vi "Get Mutation History - NONUI.vi"(6 "error in":errorcluster, 9 "Input object":refnum<class>) -> (0 "error out":errorcluster, 1 "Mutation History":T1 {"LabVIEW Version" format="%.0x"})   [LabVIEW 2019, in "IncrementMutationHistory.lvlib" / "VILIB_NONUI.lvlib"]
doc: "A mutation history is a record of all the version changes that a class has undergone and a recipie for converting flattened data of the old versions into the new version of the class. Each LabVIEW class stores its own mutation history and the mutation history for all of its ancestors. All of the mutation histories that a class records are collectively called its geneology. \n\nThis VI allows you to get a copy of the mutation history for the class or any of its ancestors. The input object is the class whose geneology you wish to search. The class name input is the mutation history that you want to find."
uses:
  <vilib>/Utility/EditLVLibs/LVClass/Mutation History.ctl
  <vilib>/Utility/EditLVLibs/LVClass/Mutation Record.ctl
  <vilib>/Utility/EditLVLibs/LibVersion.ctl
  VILIB_NONUI.lvlib
  <vilib>/Utility/EditLVLibs/Edit LVLibs.lvlib
panel:
  in  "error message 2":string="LabVIEW Object does not have mutation history for any class."
  in  "error message 1":string="The class library of the input object does not have any mutation history."
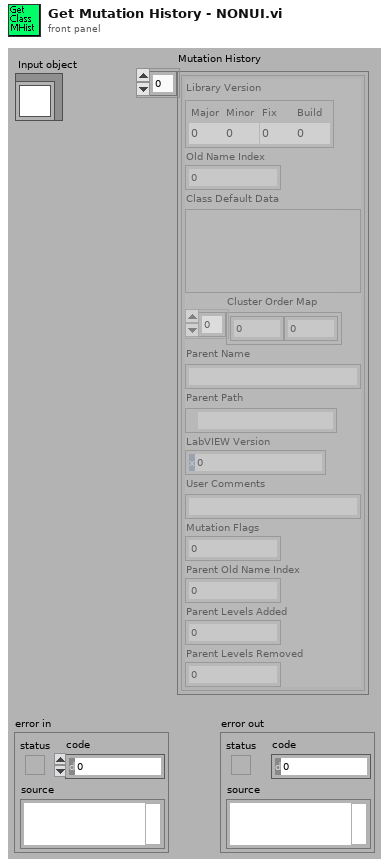
[diagram p1: front panel]
types:
  T1 = typedef "Edit LVLibs.lvlib/Mutation History.ctl" = T2[]
  T2 = typedef "Edit LVLibs.lvlib/Mutation Record.ctl" = cluster{"Library Version":T3, "Old Name Index":u8, "Class Default Data":variant, "Cluster Order Map":u32[], "Parent Name":string, "Parent Path":path, "LabVIEW Version":u32, "User Comments":string, "Mutation Flags":u8, "Parent Old Name Index":u8, "Parent Levels Added":u16, "Parent Levels Removed":u16}
  T3 = typedef "Edit LVLibs.lvlib/LibVersion.ctl" = cluster{"Major":u16, "Minor":u16, "Fix":u16, "Build":u16}
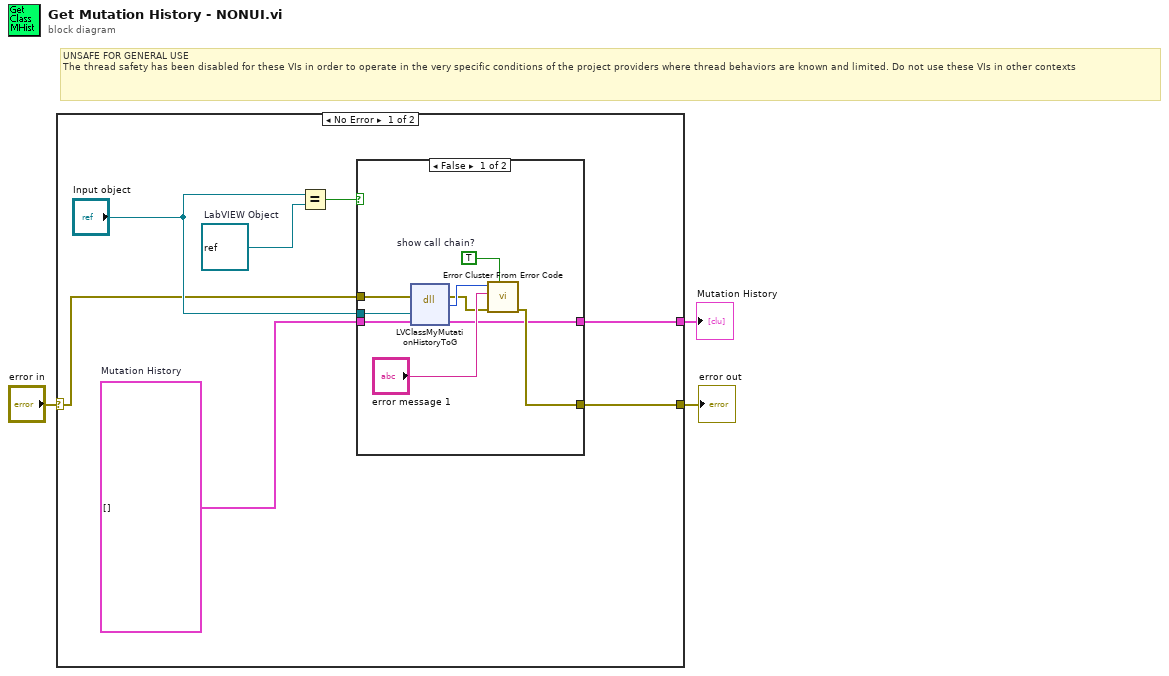
[diagram p0: block diagram]
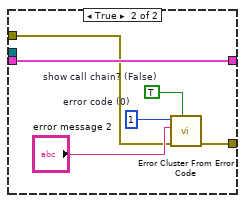
[diagram p2: hidden frame]
diagram:
  # "UNSAFE FOR GENERAL USE\nThe thread safety has been disabled for these VIs in order to operate in the very specific conditions of the project providers where thread behaviors are known and limited. Do not use these VIs in other contexts"
  n1 = case shown="No Error" "error in" {
    selector: "error in" -> [w4 w26]
    tunnel: [w7 w26] -> w3
    tunnel: [w6 _] -> w1
    frame No Error {
      w5 = refnum<class> refnum  # LabVIEW Object
      w10 = T1 []  # Mutation History
      n2 = Equal?(x="Input object", y=w5) -> (x = y?=w8:bool)
      n3 = case shown="False" w8 {
        tunnel: w10 -> [w15 w25]
        tunnel: [w14 w25] -> w6
        tunnel: "Input object" -> [w16 _]
        tunnel: [w17 w21] -> w7
        tunnel: w4 -> [w11 w20]
        frame False {
          w19 = TRUE  # show call chain?
          n4 = dll-call lib="LabVIEW" fn="LVClassMyMutationHistoryToG"(error in=w11, "object"=w16, "mutation records"=w15) -> (error out=w12:errorcluster, "return type"=w13:i32, "mutation records"=w14:T1)  [unwired: 3 in, 1 out]
          n5 = call <vilib>:"Error Cluster From Error Code.vi"("show call chain? (False)"=w19, "error in (no error)"=w12, "error message (\"\")"="error message 1", "error code (0)"=w13) -> ("error out"=w17:errorcluster)  [unwired: 5 in]
        }
        frame True {
          w23 = 1  # error code (0)
          w24 = TRUE  # show call chain? (False)
          n6 = call <vilib>:"Error Cluster From Error Code.vi"("show call chain? (False)"=w24, "error in (no error)"=w20, "error message (\"\")"="error message 2", "error code (0)"=w23) -> ("error out"=w21:errorcluster)  [unwired: 5 in]
        }
      }
    }
    frame Error {
    }
  }
  "error out" <- w3
  "Mutation History" <- w1
